vi "RT Main_test.vi"() -> ()   [LabVIEW 2017]
doc: "This template is for the Queued Message Handler design pattern.\n\nThe Event Handling Loop generates messages based on user interface actions.\n\nThe Message Handling Loop processes messages generated by the Event Handling Loop, or by other messages. The messages are string values, so new messages can be added easily to the Message Cases case structure in the Message Handling Loop. Each message cluster can also provide an optional value for Message Data, which is a variant that can be converted to whatever message-specific data is required."
uses:
  controls/FPGA State.ctl
  controls/Chatter data.ctl
  Globals/Global - All RT Loop Stop.vi
  <vilib>/rvi/errors/niLvFpgaAdjustHostInterfaceError.vi
  Globals/Global - Configuration Options.vi
  Globals/Global - RT Stream Connections.vi
  <vilib>/rvi/interface/nirviReadWriteControl/nirviReadWriteControl.xnode
  UI Error Handlers/support/Message Queue/Message Queue.lvlib
  NiFpgaLv.dll
  <vilib>/rvi/interface/Simulation/niFpgaSimulationCallBeginRW.vi
  <vilib>/nisyscfg/nisyscfg.lvlib
panel:
  out "G1 status":cluster{"G1 ":bool}
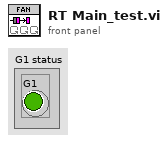
[diagram p1: front panel]
types:
  T1 = typedef "Acceleration RT FIFO Reference.ctl" = refnum<k33>
  T2 = typedef "FPGA State.ctl" = enum16{"Safe State", "Control (PID)"}
  T3 = typedef "Chatter data.ctl" = cluster{"Tool data":cluster{"Number of teeth":sgl}, "Cutting data":cluster{"rpm":sgl}, "Limits":cluster{"Magnitude threshold":sgl, "Tolerance":sgl}, "G1 status":cluster{"G1 ":bool}}
  T4 = cluster{"FPGA State":T2, "Max Acceleration Threshold":sgl, "Chatter Data":T3}
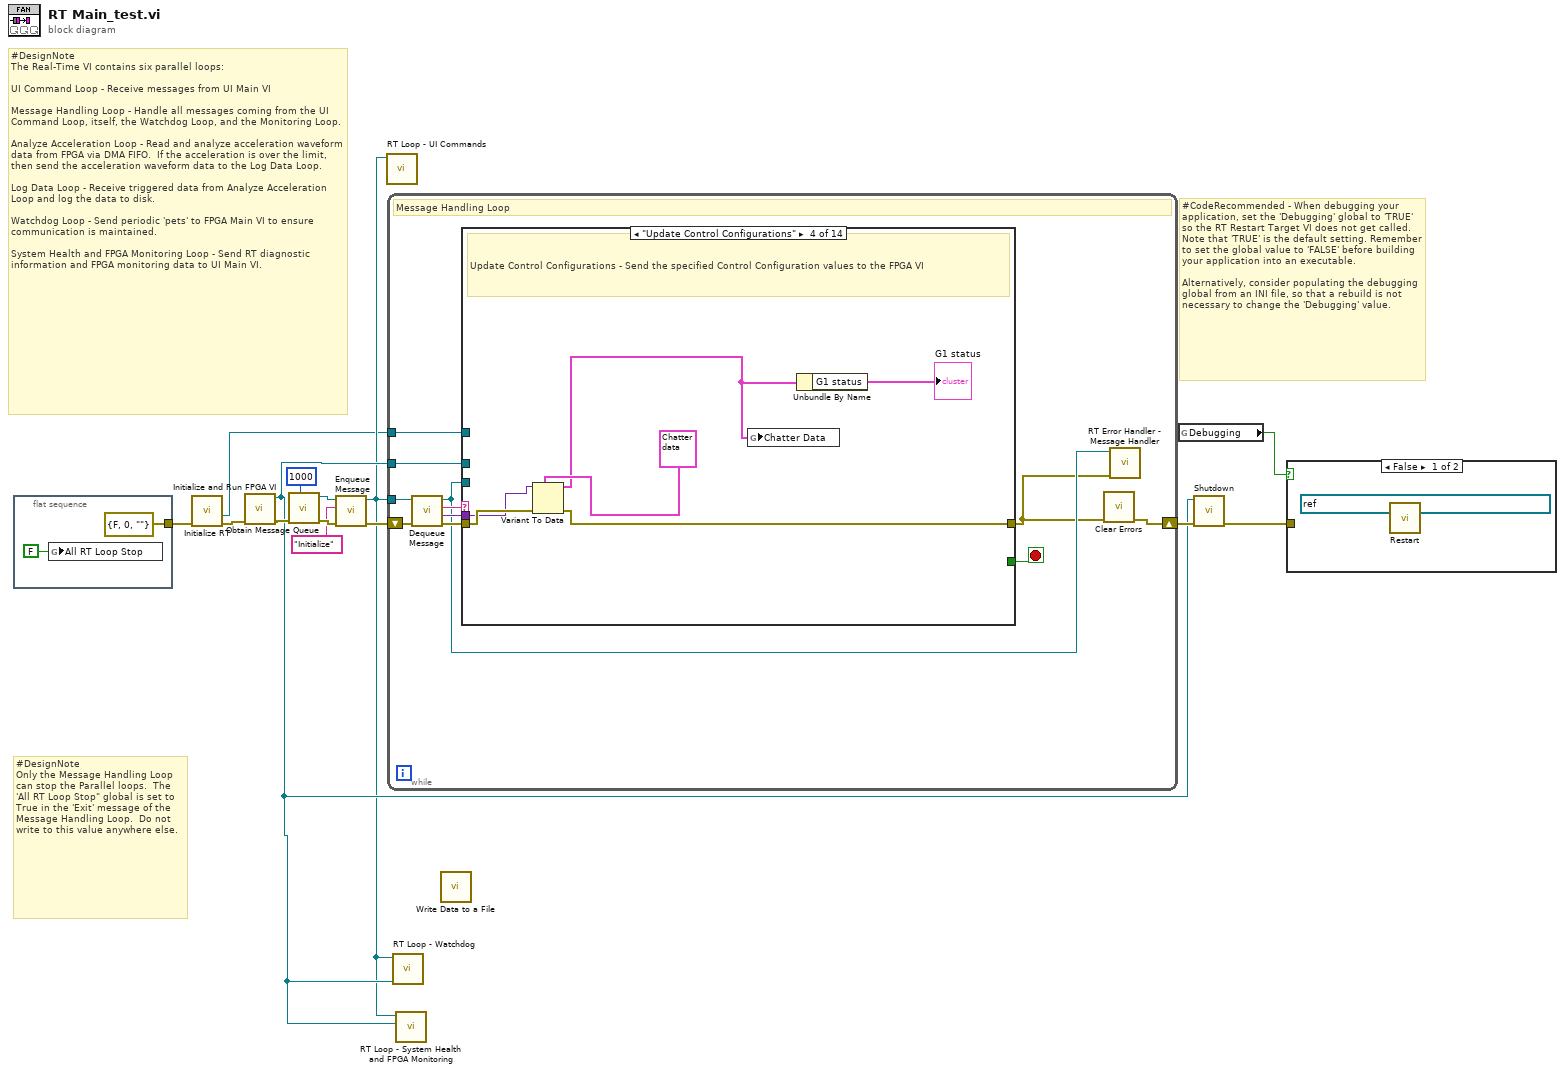
[diagram p0: block diagram]
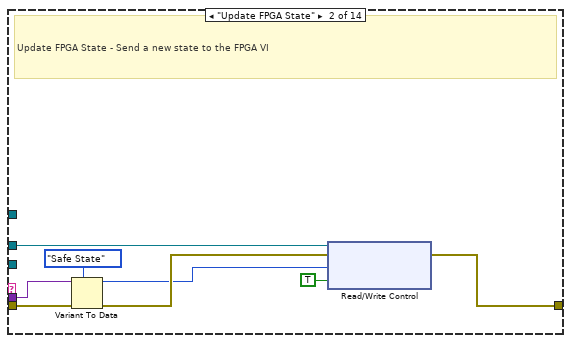
[diagram p4: hidden frame]
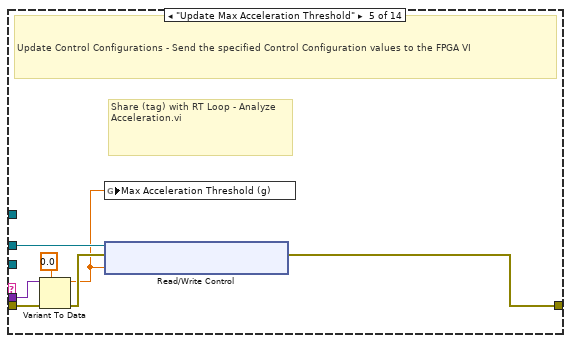
[diagram p6: hidden frame]
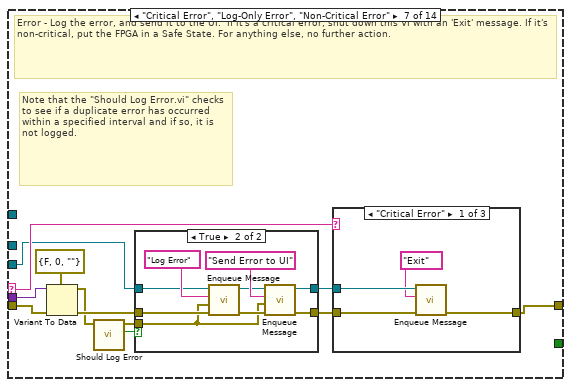
[diagram p8: hidden frame]
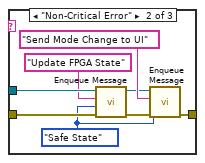
[diagram p10: hidden frame]
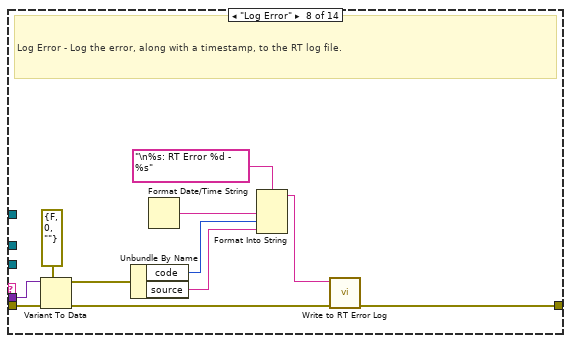
[diagram p12: hidden frame]
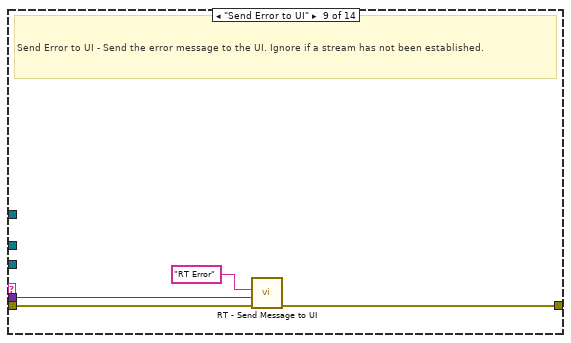
[diagram p13: hidden frame]
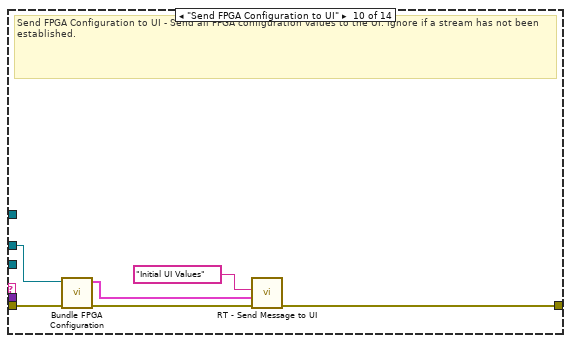
[diagram p14: hidden frame]
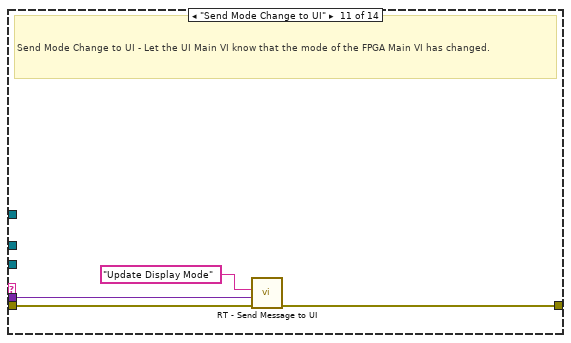
[diagram p15: hidden frame]
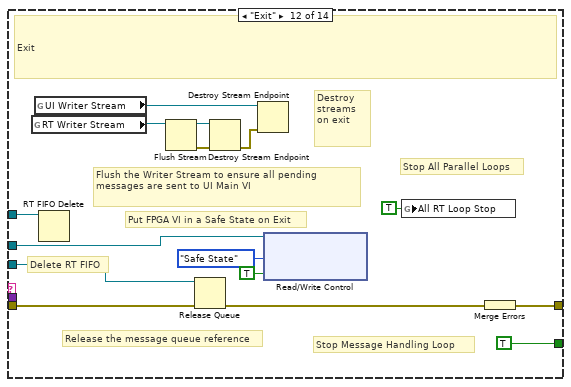
[diagram p16: hidden frame]
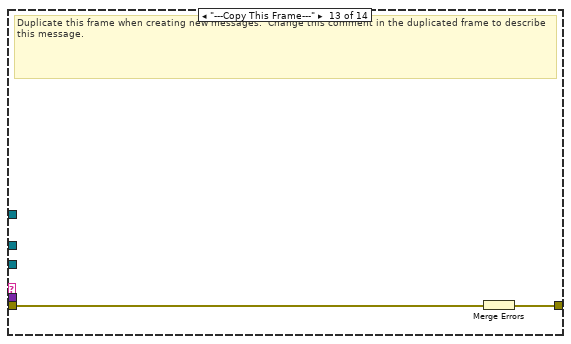
[diagram p17: hidden frame]
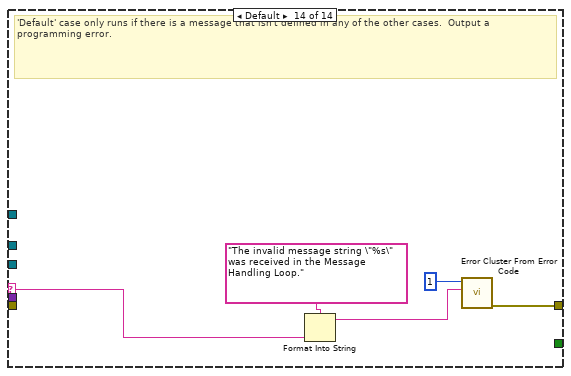
[diagram p18: hidden frame]
diagram:
  # "#CodeRecommended - When debugging your application, set the 'Debugging' global to 'TRUE' so the RT Restart Target VI does not get called.  Note that 'TRUE' is the default setting. Remember to set the global value to 'FALSE' before building your application into an executable.\n\nAlternatively, consider populating the debugging global from an INI file, so that a rebuild is not necessary to change the 'Debugging' value."
  # "#DesignNote\nThe Real-Time VI contains six parallel loops:\n\nUI Command Loop - Receive messages from UI Main VI\n\nMessage Handling Loop - Handle all messages coming from the UI Command Loop, itself, the Watchdog Loop, and the Monitoring Loop.\n\nAnalyze Acceleration Loop - Read and analyze acceleration waveform data from FPGA via DMA FIFO.  If the acceleration is over the limit, then send the acceleration waveform data to the Log Data Loop.\n\nLog Data Loop - Receive triggered data from Analyze Acceleration Loop and log the data to disk.\n\nWatchdog Loop - Send periodic 'pets' to FPGA Main VI to ensure communication is maintained.\n\nSystem Health and FPGA Monitoring Loop - Send RT diagnostic information and FPGA monitoring data to UI Main VI."
  # "#DesignNote\nOnly the Message Handling Loop can stop the Parallel loops.  The 'All RT Loop Stop\" global is set to True in the 'Exit' message of the Message Handling Loop.  Do not write to this value anywhere else."
  n1 = flat-sequence {
    tunnel: [errorcluster {"status"=FALSE, "code"=0, "source"=""} ("error constant")] -> w6
    frame #0 {
      n2 = global write "Global - All RT Loop Stop.vi" "All RT Loop Stop"(FALSE) -> ()
    }
  }
  n3 = call "Initialize RT.vi"("error in"=w6) -> ("error out"=w7:errorcluster, "Acceleration RT FIFO"=w1:T1)  [unwired: 8 in, 1 out]
  n4 = call "Initialize and Run FPGA VI.vi"("error in (no error)"=w7) -> ("error out"=w10:errorcluster, "FPGA VI Reference Out 2"=w3:refnum<k20>)  [unwired: 9 in]
  n5 = call "Obtain Message Queue.vi"("max queue size (-1, unlimited)"=1000, "error in (no error)"=w10) -> ("error out"=w14:errorcluster, "Message Queue"=w13:refnum<queue>)  [unwired: 8 in]
  n6 = call "Enqueue Message.vi"("error in (no error)"=w14, "Message"="Initialize", "Message Queue"=w13) -> ("error out"=w11:errorcluster, "dup Message Queue"=w2:refnum<queue>)  [unwired: 7 in]
  n7 = call "RT Loop - UI Commands.vi"("Message Queue"=w2) -> ()  [unwired: 11 in]
  n8 = while {
    tunnel: w2 -> [w22]
    shift-right: [w19] -> w5
    shift-left: w11 -> [w26]
    tunnel: w3 -> [w21]
    tunnel: w1 -> [w17]
    stop <- w27 stop-if-true
    # "Message Handling Loop"
    n9 = call "Dequeue Message.vi"("error in (no error)"=w26, "Message Queue"=w22) -> ("error out"=w25:errorcluster, "Message Data"=w23:variant, "Message"=w24:string, "dup Message Queue"=w20:refnum<queue>)  [unwired: 6 in]
    n10 = case "Message Cases" shown="\"Update Control Configurations\"" w24 {
      selector: w24 -> [_ _ _ _ _ _ w61 _ _ _ _ _ _ w133]
      tunnel: w20 -> [_ _ _ _ _ _ w55 _ _ _ _ w127 _ _]
      tunnel: w25 -> [w28 w36 w37 w43 w50 w51 w59 w98 w102 w108 w112 w123 w129 _]
      tunnel: [w28 w33 w37 w42 w44 w51 w60 w89 w99 w105 w111 w124 w128 w131] -> w18
      tunnel: [_ _ _ _ _ _ _ _ _ _ _ TRUE _ _] -> w27
      tunnel: w23 -> [_ w35 _ w41 w49 _ w58 w97 w101 _ w110 _ _ _]
      tunnel: w21 -> [_ w31 _ _ w47 _ _ _ _ w104 _ w119 _ _]
      tunnel: w17 -> [_ _ _ _ _ _ _ _ _ _ _ w113 _ _]
      frame "Initialize" {
        # "Initialize - Currently a no-op for the RT Main VI"
      }
      frame "Update FPGA State" {
        # "Update FPGA State - Send a new state to the FPGA VI"
        n11 = Variant To Data(error in=w36, type=FPGA_State."Safe State" ("FPGA State"), Variant=w35) -> (data=w30:T2, error out=w32:errorcluster)
        n12 = xnode "Read/Write Control"("FPGA VI Reference In"=w31, "error in"=w32, "New FPGA State"=w30, "Change State"=TRUE) -> ("error out"=w33:errorcluster)  [unwired: 1 out]
      }
      frame "Update Setpoints" {
        # "Update Setpoints - Send the specified setpoint values to the FPGA VI"
      }
      frame "Update Control Configurations" {
        # "Update Control Configurations - Send the specified Control Configuration values to the FPGA VI"
        n13 = Variant To Data(error in=w43, type=T3 {"Tool data"={"Number of teeth"=2.0}, "Cutting data"={"rpm"=9898.0}, "Limits"={"Magnitude threshold"=0.0, "Tolerance"=1.0}, "G1 status"={"G1 "=FALSE}} ("Chatter Data"), Variant=w41) -> (data=w39:T3, error out=w42:errorcluster)
        n14 = global write "Global - Configuration Options.vi" "Chatter Data"(w39) -> ()
        n15 = Unbundle By Name(w39) -> ("G1 status"=→"G1 status":cluster{"G1 ":bool})
      }
      frame "Update Max Acceleration Threshold" {
        # "Share (tag) with RT Loop - Analyze Acceleration.vi"
        # "Update Control Configurations - Send the specified Control Configuration values to the FPGA VI"
        n16 = Variant To Data(error in=w50, type=sgl 0.0 ("SGL"), Variant=w49) -> (data=w45:sgl, error out=w48:errorcluster)
        n17 = global write "Global - Configuration Options.vi" "Max Acceleration Threshold (g)"(w45) -> ()
        n18 = xnode "Read/Write Control"("FPGA VI Reference In"=w47, "error in"=w48, "Max Acceleration Threshold (g)"=w45) -> ("error out"=w44:errorcluster)  [unwired: 1 out]
      }
      frame "Update Max Fan Speed Threshold" {
        # "Update Control Configurations - Send the specified Control Configuration values to the FPGA VI"
      }
      frame "Critical Error", "Log-Only Error", "Non-Critical Error" {
        # "Note that the \"Should Log Error.vi\" checks to see if a duplicate error has occurred within a specified interval and if so, it is not logged."
        # "Error - Log the error, and send it to the UI.  If it's a critical error, shut down this VI with an 'Exit' message. If it's non-critical, put the FPGA in a Safe State. For anything else, no further action."
        n19 = Variant To Data(error in=w59, type=errorcluster {"status"=FALSE, "code"=0, "source"=""} ("error out"), Variant=w58) -> (data=w53:errorcluster, error out=w56:errorcluster)
        n20 = call "Should Log Error.vi"("error to report"=w53) -> ("Should Log Error?"=w54:bool, "dup error to report"=w52:errorcluster)  [unwired: 9 in]
        n21 = case shown="True" w54 {
          tunnel: [w65 w72] -> w63
          tunnel: [w64 w71] -> w62
          tunnel: w55 -> [w64 w70]
          tunnel: w56 -> [w65 w67]
          tunnel: w52 -> [_ w66]
          frame False {
          }
          frame True {
            n22 = call "Enqueue Message.vi"("error in (no error)"=w67, "Message Data"=w66, "Message"="Log Error", "Message Queue"=w70) -> ("error out"=w68:errorcluster, "dup Message Queue"=w69:refnum<queue>)  [unwired: 6 in]
            n23 = call "Enqueue Message.vi"("error in (no error)"=w68, "Message Data"=w66, "Message"="Send Error to UI", "Message Queue"=w69) -> ("error out"=w72:errorcluster, "dup Message Queue"=w71:refnum<queue>)  [unwired: 6 in]
          }
        }
        n24 = case shown="\"Critical Error\"" w61 {
          tunnel: w63 -> [w78 w86 w87]
          tunnel: w62 -> [w76 w85 _]
          tunnel: [w77 w82 w87] -> w60
          frame "Critical Error" {
            n25 = call "Enqueue Message.vi"("error in (no error)"=w78, "Message"="Exit", "Message Queue"=w76) -> ("error out"=w77:errorcluster)  [unwired: 7 in, 1 out]
          }
          frame "Non-Critical Error" {
            w79 = FPGA_State."Safe State" ("FPGA State")
            n26 = call "Enqueue Message.vi"("error in (no error)"=w86, "Message Data"=w79, "Message"="Update FPGA State", "Message Queue"=w85) -> ("error out"=w83:errorcluster, "dup Message Queue"=w80:refnum<queue>)  [unwired: 6 in]
            n27 = call "Enqueue Message.vi"("error in (no error)"=w83, "Message Data"=w79, "Message"="Send Mode Change to UI", "Message Queue"=w80) -> ("error out"=w82:errorcluster)  [unwired: 6 in, 1 out]
          }
          frame Default {
          }
        }
      }
      frame "Log Error" {
        # "Log Error - Log the error, along with a timestamp, to the RT log file."
        n28 = Variant To Data(error in=w98, type=errorcluster {"status"=FALSE, "code"=0, "source"=""} ("error constant"), Variant=w97) -> (data=w92:errorcluster, error out=w95:errorcluster)
        n29 = Unbundle By Name(w92) -> ("code"=w91:i32, "source"=w90:string)
        n30 = Format Date/Time String() -> (date/time string=w93:string)  [unwired: 3 in]
        n31 = Format Into String(format string="\n%s: RT Error %d - %s", w93, w91, w90) -> (resulting string=w88:string)  [unwired: 2 in, 1 out]
        n32 = call "Write to RT Error Log.vi"("error in (no error)"=w95, "Log Entry"=w88) -> ("error out"=w89:errorcluster)  [unwired: 9 in]
      }
      frame "Send Error to UI" {
        # "Send Error to UI - Send the error message to the UI. Ignore if a stream has not been established."
        n33 = call "RT - Send Message to UI.vi"("error in (no error)"=w102, "Message Data"=w101, "Message"="RT Error") -> ("error out"=w99:errorcluster)  [unwired: 8 in]
      }
      frame "Send FPGA Configuration to UI" {
        # "Send FPGA Configuration to UI - Send all FPGA configuration values to the UI. Ignore if a stream has not been established."
        n34 = call "Bundle FPGA Configuration.vi"("error in (no error)"=w108, "FPGA VI Reference Out 2"=w104) -> ("error out"=w107:errorcluster, "Cluster"=w103:T4)  [unwired: 8 in]
        n35 = call "RT - Send Message to UI.vi"("error in (no error)"=w107, "Message Data"=w103, "Message"="Initial UI Values") -> ("error out"=w105:errorcluster)  [unwired: 8 in]
      }
      frame "Send Mode Change to UI" {
        # "Send Mode Change to UI - Let the UI Main VI know that the mode of the FPGA Main VI has changed."
        n36 = call "RT - Send Message to UI.vi"("error in (no error)"=w112, "Message Data"=w110, "Message"="Update Display Mode") -> ("error out"=w111:errorcluster)  [unwired: 8 in]
      }
      frame "Exit" {
        # "Delete RT FIFO"
        # "Flush the Writer Stream to ensure all pending messages are sent to UI Main VI"
        # "Destroy streams on exit"
        # "Put FPGA VI in a Safe State on Exit"
        # "Stop Message Handling Loop"
        # "Stop All Parallel Loops"
        # "Release the message queue reference"
        # "Exit"
        n37 = global read "Global - RT Stream Connections.vi" "RT Writer Stream"() -> (w116:refnum<k21>)
        n38 = global read "Global - RT Stream Connections.vi" "UI Writer Stream"() -> (w118:refnum<k21>)
        n39 = RT FIFO Delete(0:w113) -> ()  [unwired: 2 in, 1 out]
        n40 = Flush Stream(11:w116) -> (0:w114:errorcluster, 3:w115:refnum<k21>)  [unwired: 3 in, 1 out]
        n41 = Release Queue(queue=w127, error in (no error)=w123) -> (error out=w125:errorcluster)  [unwired: 1 in, 2 out]
        n42 = Destroy Stream Endpoint(8:w114, 11:w115) -> (0:w117:errorcluster)
        n43 = Destroy Stream Endpoint(8:w117, 11:w118) -> ()  [unwired: 1 out]
        n44 = xnode "Read/Write Control"("FPGA VI Reference In"=w119, "New FPGA State"=FPGA_State."Safe State" ("New State"), "Change State"=TRUE) -> ()  [unwired: 1 in, 2 out]
        n45 = global write "Global - All RT Loop Stop.vi" "All RT Loop Stop"(TRUE ("Stop Monitoring Loops")) -> ()
        n46 = Merge Errors(w125) -> (w124:errorcluster)
      }
      frame "---Copy This Frame---" {
        # "Duplicate this frame when creating new messages.  Change this comment in the duplicated frame to describe this message."
        n47 = Merge Errors(w129) -> (w128:errorcluster)
      }
      frame Default {
        # "'Default' case only runs if there is a message that isn't defined in any of the other cases.  Output a programming error."
        n48 = Format Into String(format string="The invalid message string \"%s\" was received in the Message Handling Loop." ("Unknown Message Error Text"), w133) -> (resulting string=w130:string)  [unwired: 2 in, 1 out]
        n49 = call <vilib>:"Error Cluster From Error Code.vi"("error message (\"\")"=w130, "error code (0)"=1) -> ("error out"=w131:errorcluster)  [unwired: 7 in]
      }
    }
    n50 = call <vilib>:"Clear Errors.vi"("error in (no error)"=w18) -> ("error out"=w19:errorcluster)  [unwired: 5 in, 1 out]
    n51 = call "RT Error Handler - Message Handler.vi"("error in (no error)"=w18, "Message Queue"=w20) -> ()  [unwired: 9 in, 1 out]
  }
  n52 = call "RT Loop - Watchdog.vi"("FPGA VI Reference in"=w3, "Message Queue"=w2) -> ()  [unwired: 10 in]
  n53 = call "RT Loop - System Health and FPGA Monitoring.vi"("FPGA VI Reference Out 2"=w3, "Message Queue"=w2) -> ()  [unwired: 9 in, 1 out]
  n54 = call "Write Data to a File.vi"() -> ()  [unwired: 12 in]
  n55 = global read "Global - Configuration Options.vi" "Debugging"() -> (w9:bool)
  n56 = call "Shutdown.vi"("error in"=w5, "FPGA VI Reference in"=w3) -> ("error out"=w4:errorcluster)  [unwired: 9 in]
  n57 = case shown="False" w9 {
    tunnel: w4 -> [_ _]
    frame False {
      n58 = call <vilib>:"Restart.vi"("Session in"=refnum<k21> "NI-cRIO-9045-01DAA691 (143.167.159.188)" ("session in")) -> ()  [unwired: 8 in, 3 out]
    }
    frame True {
    }
  }
